vi "Pre Launch Init.vi"(11 "Preparation Line in":refnum<class "Preparation Line.lvclass">) -> (0 "error out":errorcluster, 3 "Preparation Line out":refnum<class "Preparation Line.lvclass">)   [LabVIEW 2015, in "cRIO-Carbondioxide.lvlib" / "CO2-Actor.lvlib" / "Preparation Line.lvclass"]
doc: "(<B>Filename</B>: Actor Framework.lvlib:Actor.lvclass:Pre Launch Init.vi)\n\nDefines behavior that occurs after the Launch Actor method is invoked but before the actor's Actor Core method begins running.\n\nThe Pre Launch Init method is guaranteed to finish before the Launch Actor method returns to its caller and before the actor itself receives any messages. Any references that the Pre Launch Init method obtains are guaranteed to have the same lifetime as the actor itself. Any errors that the Pre Launch Init method returns will abort the launch.\n\nBy default, this method does nothing. A descendant class may override it to define behavior."
uses:
  Preparation Line.lvclass
  Preparation Line.lvclass/Preparation Line.ctl
  <vilib>/ActorFramework/Actor/Actor.lvclass/Actor.ctl
  <vilib>/ActorFramework/Message Enqueuer/Message Enqueuer.lvclass/Message Enqueuer.ctl
  <vilib>/ActorFramework/Actor/Read Self Enqueuer.vi
  <vilib>/ActorFramework/Message Enqueuer/Enqueue.vi
  <vilib>/ActorFramework/Message Enqueuer/Init from Existing Queue.vi
  <vilib>/ActorFramework/Message Priority Queue/Priority Enqueue.vi
  CO2 Actor/CO2 Actor.lvclass
  CO2 Actor Messages/Launch Nested Actors Msg/Launch Nested Actors Msg.lvclass
  <vilib>/ActorFramework/Message Enqueuer/Message Enqueuer.lvclass
  <vilib>/ActorFramework/Actor/Actor.lvclass
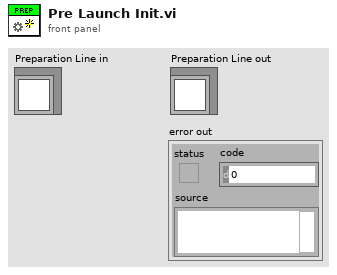
[diagram p1: front panel]
types:
  T1 = typedef "Sample Container.ctl" = cluster{"Sample In":refnum<k21>, "Sample Name":refnum<k21>, "Ti Cathode":refnum<k21>, "SampleQ":refnum<queue>}
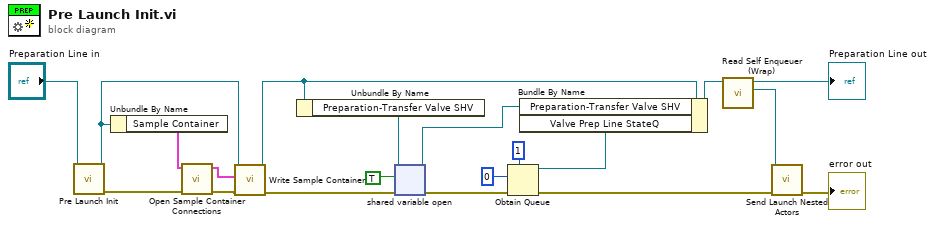
[diagram p0: block diagram]
diagram:
  n1 = call-parent "Pre Launch Init.vi"("CO2 Actor in"="Preparation Line in") -> ("error out"=w9:errorcluster, "CO2 Actor out"=w7:refnum<class "Preparation Line.lvclass">)  [unwired: 9 in]
  n2 = Unbundle By Name(w7) -> ("Sample Container"=w8:T1)
  n3 = call "Open Sample Container Connections.vi"("error in (no error)"=w9, "Container in"=w8) -> ("error out"=w19:errorcluster, "Container out"=w10:T1)  [unwired: 8 in]
  n4 = call "Write Sample Container.vi"("error in (no error)"=w19, "Sample Container"=w10, "Preparation Line in"=w7) -> ("error out"=w14:errorcluster, "Preparation Line out"=w15:refnum<class "Preparation Line.lvclass">)  [unwired: 7 in]
  n5 = Unbundle By Name(w15) -> ("Preparation-Transfer Valve SHV"=w13:refnum<k21>)
  n6 = shared-variable-open(w13, w14, TRUE) -> (w6:refnum<k21>, w5:errorcluster)  [unwired: 1 in]
  n7 = Obtain Queue(max queue size (-1, unlimited)=1, element data type=u16 0, error in (no error)=w5) -> (queue out=w3:refnum<queue>, error out=w4:errorcluster)  [unwired: 2 in, 1 out]
  n8 = Bundle By Name(cluster=w15, "Preparation-Transfer Valve SHV"=w6, "Valve Prep Line StateQ"=w3) -> (w11:refnum<class "Preparation Line.lvclass">)
  n9 = call "Read Self Enqueuer (Wrap).vi"("CO2 Actor in"=w11) -> ("Actor Framework:Message Enqueuer"=w16:refnum<class "Message Enqueuer.lvclass">, "CO2 Actor out"=→"Preparation Line out":refnum<class "Preparation Line.lvclass">)  [unwired: 9 in]
  n10 = call "Send Launch Nested Actors.vi"("error in (no error)"=w4, "Message Enqueuer"=w16) -> ("error out"=→"error out":errorcluster)  [unwired: 8 in, 1 out]
